vi "process.vi"(8 "error in":errorcluster, 9 "result allocation":T1, 10 "parameters":T1, 11 "AppStateMachine runtime in":refnum<class "AppStateMachine runtime.lvclass">) -> (0 "error out":errorcluster, 1 "results":T1, 2 "parameter allocation":T1, 3 "AppStateMachine runtime out":refnum<class "AppStateMachine runtime.lvclass">)   [LabVIEW 2017, in "AppStateMachine runtime.lvclass"]
doc: "Provides an interface for information processing by a module at runtime. While this interface performs no operations, a child should provide an override which may process data in any manner necessary."
uses:
  AppStateMachine runtime.lvclass
  <vilib>/NI/Tag Bus/table/data table.ctl
  StateId.ctl
  AppStateMachine runtime.lvclass/AppStateMachine runtime.ctl
  <vilib>/NI/NI JSONRPC Server Framework/Classes/Server/JSONRPC Server.lvclass
  <instrlib>/_niInstr/Instruction Framework/v1/Host/Instruction Target/niInstr Instruction Target v1 Host.lvclass
  <instrlib>/_niInstr/Instruction Framework/v1/Host/Instruction Framework Context/niInstr Instruction Framework Context v1 Host.lvclass
  <vilib>/NI/Tag Bus/table/data table.lvlib
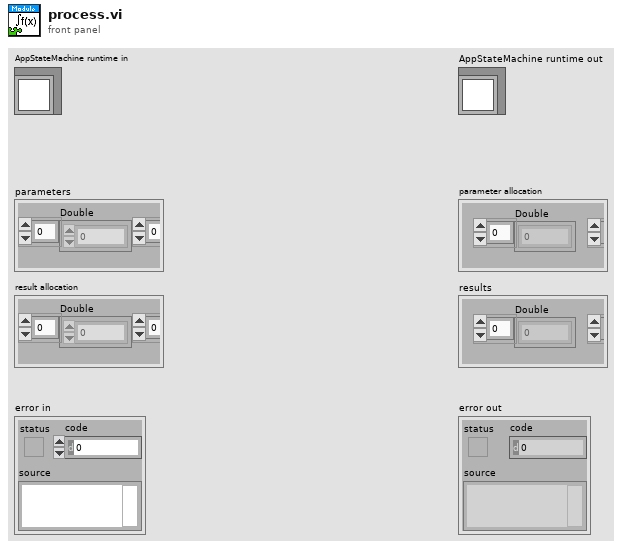
[diagram p1: front panel]
types:
  T1 = typedef "tag bus.lvlib/data table.lvlib/data table.ctl" = cluster{"Double":dbl[], "Single":sgl[], "I64":i64[], "I32":i32[], "I16":i16[], "I8":i8[], "U64":u64[], "U32":u32[], "U16":u16[], "U8":u8[], "Boolean":bool[], "String":string[], "Array of Double":cluster{"DBL Array":dbl[]}[], "Array of Single":cluster{"SGL Array":sgl[]}[], "Array of I64":cluster{"I64 Array":i64[]}[], "Array of I32":cluster{"I32 Array":i32[]}[], "Array of I16":cluster{"I16 Array":i16[]}[], "Array of I8":cluster{"I8 Array":i8[]}[], "Array of U64":cluster{"U64 Array":u64[]}[], "Array of U32":cluster{"U32 Array":u32[]}[], "Array of U16":cluster{"U16 Array":u16[]}[], "Array of U8":cluster{"U8 Array":u8[]}[], "Array of Boolean":cluster{"Boolean Array":bool[]}[], "Array of String":cluster{"String Array":string[]}[]}
  T2 = typedef "AppStateMachine runtime.lvclass/StateId.ctl" = enum16{"Initialize", "Idle", "TunePLL", "TuneAFE", "TuneBuckBoost", "Precharge", "Synchronize", "Ready", "EnableAFE", "EnableBuckBoost", "Powered", "SafeState", "UnrecoverableSafeState"}
  T3 = typedef "AppStateMachine configuration.lvclass/parameter data indices.ctl" = cluster{"Double.CPU":i32, "Double.Memory":i32, "Double.Disk":i32}
  T4 = typedef "AppStateMachine configuration.lvclass/result data indices.ctl" = cluster{"U16.State":i32, "Boolean.LED_Enable":i32, "I32.LED_BlinksPerCycle":i32, "Boolean.LED_GreenOrYellow":i32}
  T5 = typedef "AppStateMachine runtime.lvclass/Interfaces.ctl" = cluster{"FPGA Ref":T6, "RPC_Server":refnum<class "JSONRPC Server.lvclass">, "ThreePhasePLL":T7, "ActiveFrontEnd":T8, "BuckBoost":T9}
  T6 = typedef "AppStateMachine runtime.lvclass/FPGAtypedef.ctl" = refnum<k20>
  T7 = typedef "ThreePhasePLLInterface.lvlib/InterfaceRef.ctl" = cluster{"instruction target":refnum<class "niInstr Instruction Target v1 Host.lvclass">, "context":refnum<class "niInstr Instruction Framework Context v1 Host.lvclass">}
  T8 = typedef "AFE_interface.lvlib/InterfaceRef.ctl" = cluster{"instruction target":refnum<class "niInstr Instruction Target v1 Host.lvclass">, "context":refnum<class "niInstr Instruction Framework Context v1 Host.lvclass">}
  T9 = typedef "BuckBoostInterface.lvlib/Interface.ctl" = cluster{"instruction target":refnum<class "niInstr Instruction Target v1 Host.lvclass">, "BuckBoostContext":refnum<class "niInstr Instruction Framework Context v1 Host.lvclass">}
  T10 = typedef "AppStateMachine runtime.lvclass/State.ctl" = cluster{"StateId":T2, "LED_Enable":bool, "LED_BlinksPerCycle":i32, "LED_Color":T11, "ResourceUsage":cluster{"CPU":dbl, "Memory":dbl, "Disk":dbl}, "locked":bool, "Detected Frequency":dbl, "VDCLink":dbl, "VLoad":dbl, "Fault Registers":u64, "afeEnabled":bool, "buckboostEnabled":bool, "timer":u32, "PrechargeTimeout":u32, "SynchronizeTimeout":u32, "DCLinkSteadyState":dbl, "PrechargeLevel":dbl, "DCLinkSteadyStateTimeout":u32, "ILoad":dbl}
  T11 = typedef "AppStateMachine runtime.lvclass/LED_Color.ctl" = enum16{"Green", "Yellow"}
  T12 = typedef "AppStateMachine runtime.lvclass/parameter user data.ctl" = cluster{"CPU":dbl, "Memory":dbl, "Disk":dbl}
  T13 = typedef "AppStateMachine runtime.lvclass/methods.ctl" = enum16{"none", "echo", "GetResourceUsage", "CheckConnection", "CurrentState", "GoToSafeState", "ClearSafeState", "AvailableLogs", "ForceLogTrigger", "GoToTuneAFE", "GoToTunePLL", "GoToTuneBuckBoost", "TurnOnSystem", "TurnOffSystem", "PrechargeSystem", "SetPLL_Tune", "SetBuckBoostSetpoint", "SetAFE_tune", "SetBuckBoostTune", "CompleteTuning", "PllSettings", "AfeSettings", "BuckBoostSettings", "enableAfe", "disableAfe", "enableBuckBoost", "disableBuckBoost"}
  T14 = typedef "AppStateMachine runtime.lvclass/result user data.ctl" = cluster{"State":u16, "LED_Enable":bool, "LED_BlinksPerCycle":i32, "LED_GreenOrYellow":bool}
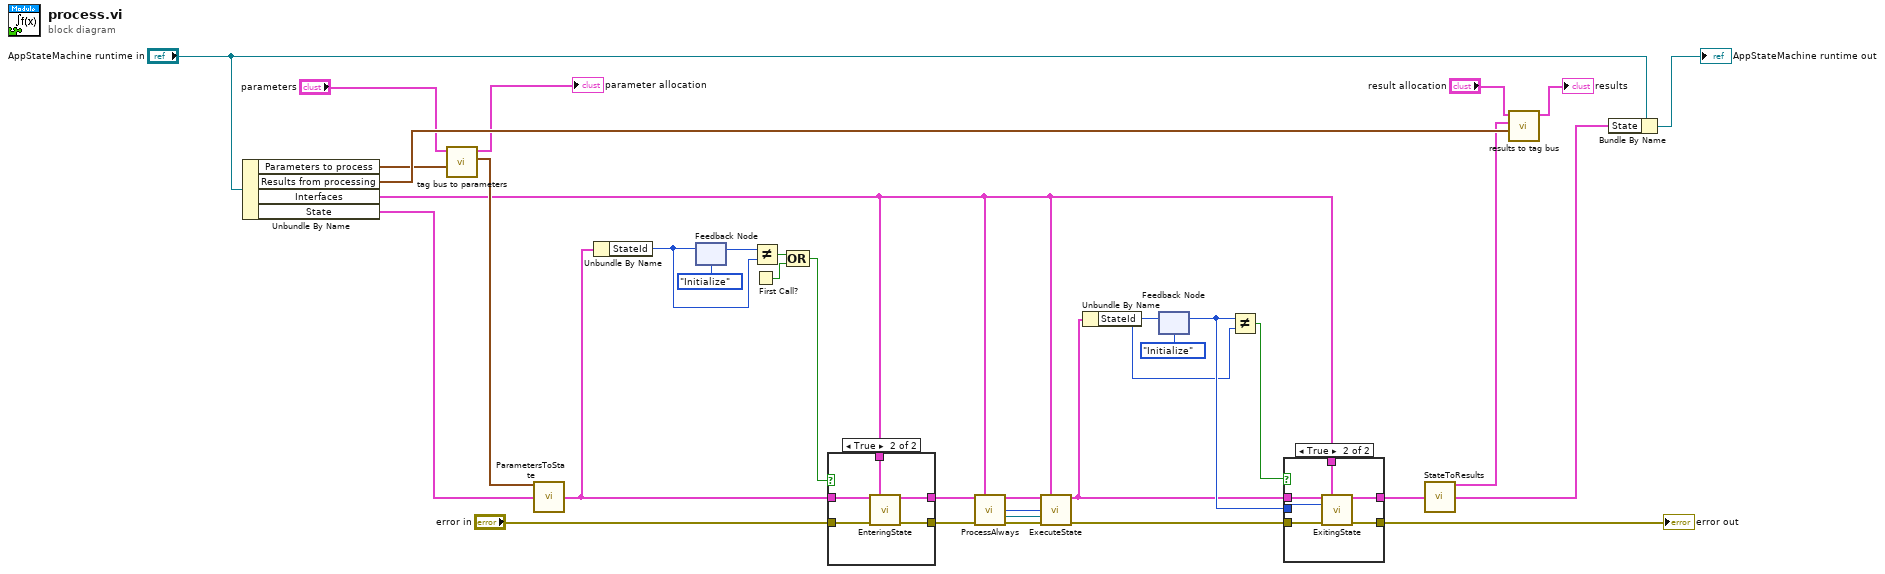
[diagram p0: block diagram]
diagram:
  n1 = Unbundle By Name("AppStateMachine runtime in") -> ("Parameters to process"=w30:T3, "Results from processing"=w33:T4, "Interfaces"=w5:T5, "State"=w17:T10)
  n2 = call "tag bus to parameters.vi"("indices"=w30, "tag bus in"="parameters") -> ("data cluster"=w18:T12, "tag bus out"=→"parameter allocation":T1)  [unwired: 8 in]
  n3 = call "ParametersToState.vi"("ParametersToState"=w18, "StateIn"=w17) -> ("StateOut"=w16:T10)  [unwired: 13 in]
  n4 = Unbundle By Name(w16) -> ("StateId"=w19:T2)
  n5 = feedback-in #1(w19) -> ()
  n6 = feedback #1(StateId."Initialize" ("State")) -> (w26:T2)
  n7 = First Call?() -> (First Call?: T/F=w9:bool)
  n8 = Not Equal?(x=w26, y=w19) -> (x != y?=w11:bool)
  n9 = Compound Arithmetic op=OR(w11, w9) -> (w10:bool)
  n10 = case shown="True" w10 {
    tunnel: "error in" -> [w37 w42]
    tunnel: w16 -> [w36 w39]
    tunnel: [w37 w41] -> w4
    tunnel: w5 -> [_ w40]
    tunnel: [w36 w38] -> w7
    frame False {
    }
    frame True {
      n11 = call "EnteringState.vi"("StateIn"=w39, "Interfaces"=w40, "error in (no error)"=w42) -> ("StateOut"=w38:T10, "error out"=w41:errorcluster)  [unwired: 11 in]
    }
  }
  n12 = call "ProcessAlways.vi"("StateIn"=w7, "Interfaces"=w5, "error in"=w4) -> ("StateOut"=w6:T10, "method"=w2:T13, "params"=w1:refnum<class "JSON Null.lvclass">, "error out"=w3:errorcluster)  [unwired: 9 in]
  n13 = call "ExecuteState.vi"("StateIn"=w6, "Interfaces"=w5, "methods"=w2, "params"=w1, "error in (no error)"=w3) -> ("StateOut"=w8:T10, "error out"=w22:errorcluster)  [unwired: 9 in]
  n14 = Unbundle By Name(w8) -> ("StateId"=w15:T2)
  n15 = feedback #2(StateId."Initialize" ("State")) -> (w21:T2)
  n16 = feedback-in #2(w15) -> ()
  n17 = Not Equal?(x=w21, y=w15) -> (x != y?=w23:bool)
  n18 = case shown="True" w23 {
    tunnel: w22 -> [w44 w50]
    tunnel: w21 -> [_ w47]
    tunnel: [w44 w49] -> w20
    tunnel: [w43 w45] -> w14
    tunnel: w5 -> [_ w48]
    tunnel: w8 -> [w43 w46]
    frame False {
    }
    frame True {
      n19 = call "ExitingState.vi"("StateIn"=w46, "Interfaces"=w48, "ExitingState"=w47, "error in (no error)"=w50) -> ("StateOut"=w45:T10, "error out"=w49:errorcluster)  [unwired: 10 in]
    }
  }
  "error out" <- w20
  n20 = call "StateToResults.vi"("StateIn"=w14) -> ("Results"=w12:T14, "StateOut"=w13:T10)  [unwired: 13 in]
  n21 = call "results to tag bus.vi"("indices"=w33, "data cluster"=w12, "tag bus in"="result allocation") -> ("tag bus out"=→"results":T1)  [unwired: 8 in]
  n22 = Bundle By Name(cluster="AppStateMachine runtime in", "State"=w13) -> (→"AppStateMachine runtime out":refnum<class "AppStateMachine runtime.lvclass">)
